vi "DataSelect.vi"(8 "error in (no error)":errorcluster, 10 "Table":string, 11 "Machine":string) -> (0 "error out":errorcluster)   [LabVIEW 2012]
uses:
  <vilib>/addons/database/Connection.llb/DB Tools Open Connec (Path).vi
  <vilib>/addons/database/_DB Variant To Data/Database Variant To Data.xnode
  <vilib>/addons/database/NI_Database_API.lvlib
panel:
  out "data 2":string
  out "element":i32
  out "x = y? 2":bool
  out "sum":i32
  out "concatenated string 2":string
  out "output cluster 2":T1
  in  "input cluster 2":T1
  out "sum 2":i32
  out "x = y?":bool
  out "output cluster":T1
  in  "input cluster":T1
  out "data":variant[][](array[variant])
  out "concatenated string":string
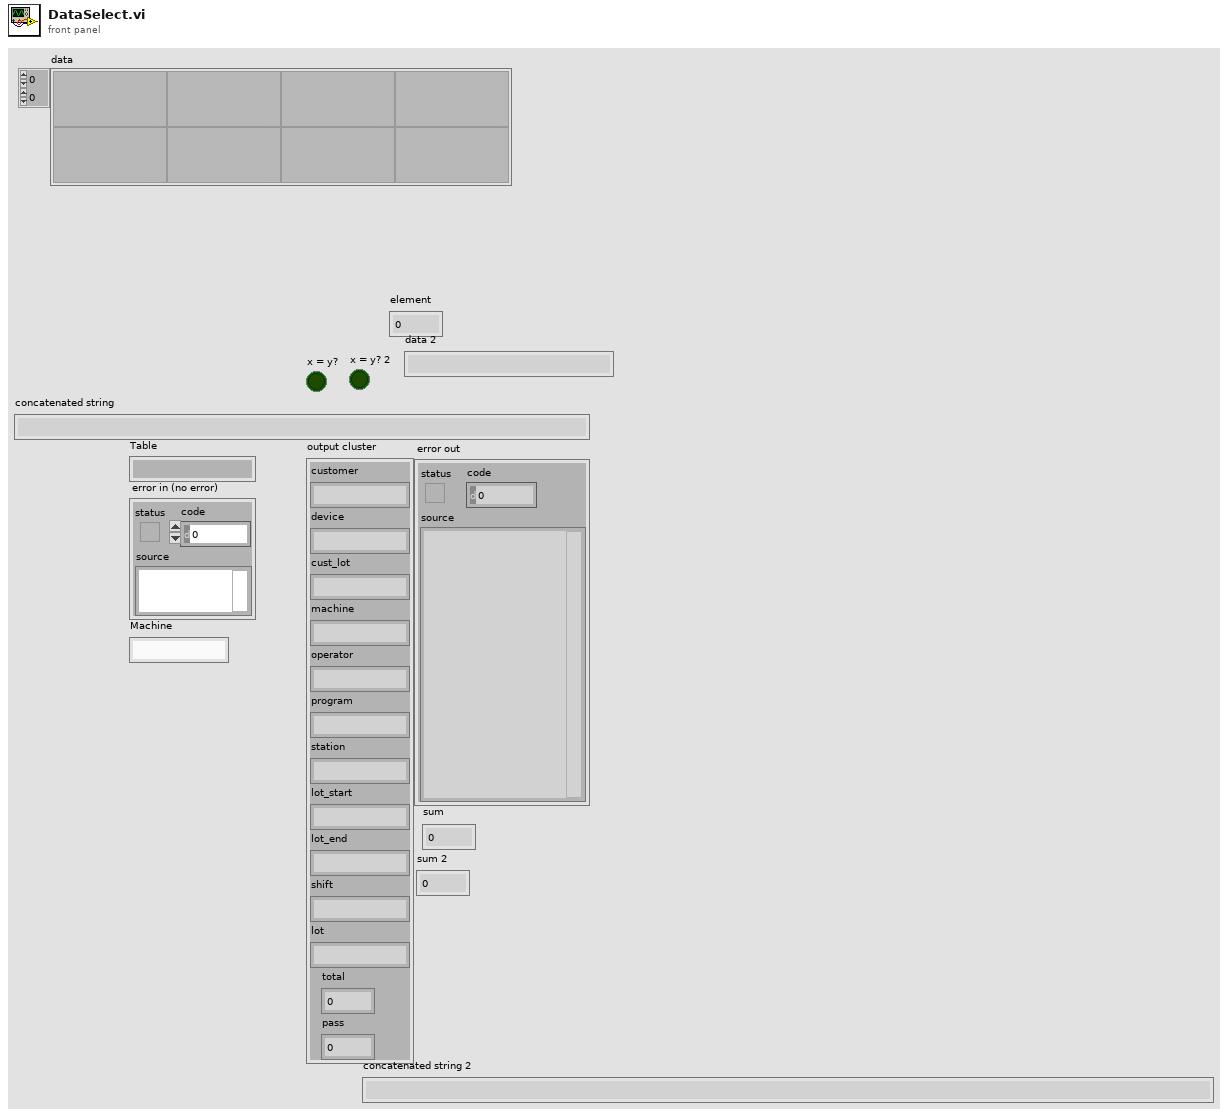
[diagram p1: front panel]
types:
  T1 = cluster{"customer":string, "device":string, "cust_lot":string, "machine":string, "operator":string, "program":string, "station":string, "lot_start":string, "lot_end":string, "shift":string, "lot":string, "total":dbl, "pass":dbl}
  T2 = typedef "NI_Database_API.lvlib/Conn ObjectReference.ctl" = refnum<k1>
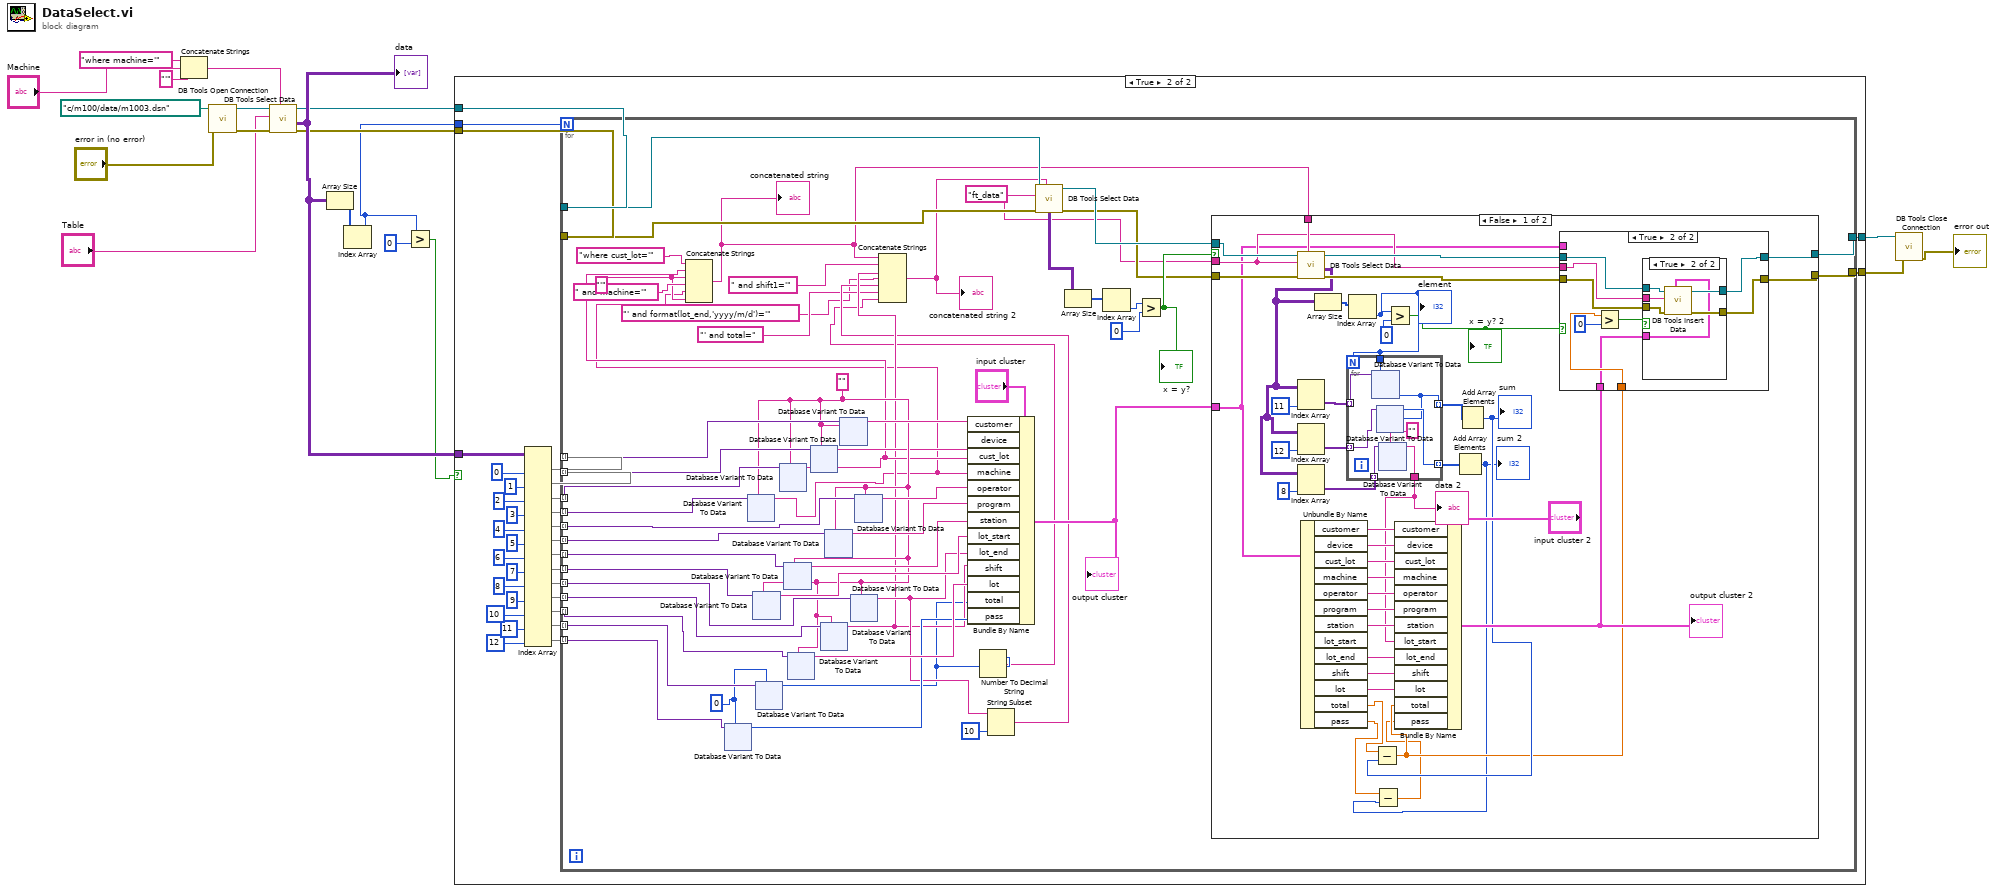
[diagram p0: block diagram]
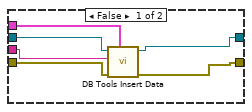
[diagram p3: hidden frame]
diagram:
  n1 = Concatenate Strings("where machine='" ("string"), "Machine", "'" ("string")) -> (w6:string)
  n2 = call-poly <vilib>:"DB Tools Open Connection.vi"("error in (no error)"="error in (no error)", "connection information"=path "c:/m100/data/m1003.dsn") -> ("error out"=w17:errorcluster, "connection reference"=w18:T2)  [unwired: 6 in]
  n3 = call <vilib>:"DB Tools Select Data.vi"("condition"=w6, "error in (no error)"=w17, "table"="Table", "connection reference"=w18) -> ("error out"=w3:errorcluster, "data"=w15:variant[][], "connection reference out"=w4:T2)  [unwired: 2 in]
  "data" <- w15
  n4 = Array Size(array=w15) -> (size(s)=w16:i32[])
  n5 = Index Array(array=w16) -> (element=w2:i32)  [unwired: 1 in]
  n6 = Greater?(x=w2, y=0) -> (0:w1:bool)
  n7 = case shown="True" w1 {
    tunnel: w15 -> [_ w52]
    tunnel: [w21 w26] -> w14
    tunnel: [w20 w25] -> w13
    tunnel: w4 -> [w21 w24]
    tunnel: w3 -> [w20 w23]
    tunnel: w2 -> [_ w22]
    frame False {
    }
    frame True {
      n8 = Index Array(array=w52, index (col) #1=0 ("disabled index (col)"), index (col) #2=1 ("index (col)"), index (col) #3=2 ("index (col)"), index (col) #4=3 ("index (col)"), index (col) #5=4 ("index (col)"), index (col) #6=5 ("index (col)"), index (col) #7=6 ("index (col)"), index (col) #8=7 ("index (col)"), index (col) #9=8 ("index (col)"), index (col) #10=9 ("index (col)"), index (col) #11=10 ("index (col)"), index (col) #12=11 ("index (col)"), index (col) #13=12 ("index (col)")) -> (element #1=w39:variant[], element #2=w38:variant[], element #3=w37:variant[], element #4=w36:variant[], element #5=w35:variant[], element #6=w34:variant[], element #7=w33:variant[], element #8=w32:variant[], element #9=w31:variant[], element #10=w30:variant[], element #11=w29:variant[], element #12=w28:variant[], element #13=w27:variant[])  [unwired: 13 in]
      n9 = for {
        N: w22 -> [_]
        tunnel: w24 -> [w83]
        tunnel: w23 -> [w82]
        tunnel: w39 -> [w105] mode=indexing
        tunnel: w38 -> [w104] mode=indexing
        tunnel: w37 -> [w103] mode=indexing
        tunnel: w36 -> [w102] mode=indexing
        tunnel: w35 -> [w92] mode=indexing
        tunnel: w34 -> [w101] mode=indexing
        tunnel: w33 -> [w100] mode=indexing
        tunnel: w32 -> [w99] mode=indexing
        tunnel: w31 -> [w98] mode=indexing
        tunnel: w30 -> [w97] mode=indexing
        tunnel: w29 -> [w96] mode=indexing
        tunnel: w28 -> [w95] mode=indexing
        tunnel: w27 -> [w94] mode=indexing
        tunnel: [w71] -> w26
        tunnel: [w70] -> w25
        w56 = "'" ("string")
        w73 = "ft_data" ("table")
        w93 = 0
        w79 = ""
        n10 = xnode "Database Variant To Data"("database variant"=w94, "type"=w93) -> ("data"=w85:i32)  [unwired: 1 in, 1 out]
        n11 = xnode "Database Variant To Data"("database variant"=w102, "type"=w79) -> ("data"=w55:string)  [unwired: 1 in, 1 out]
        n12 = xnode "Database Variant To Data"("database variant"=w99, "type"=w79) -> ("data"=w87:string)  [unwired: 1 in, 1 out]
        n13 = xnode "Database Variant To Data"("database variant"=w95, "type"=w93) -> ("data"=w61:i32)  [unwired: 1 in, 1 out]
        n14 = xnode "Database Variant To Data"("database variant"=w103, "type"=w79) -> ("data"=w67:string)  [unwired: 1 in, 1 out]
        n15 = Concatenate Strings("where cust_lot='" ("string"), w67, w56, " and machine='" ("string"), w55, w56) -> (w54:string)
        "concatenated string" <- w54
        n16 = xnode "Database Variant To Data"("database variant"=w100, "type"=w79) -> ("data"=w88:string)  [unwired: 1 in, 1 out]
        n17 = xnode "Database Variant To Data"("database variant"=w96, "type"=w79) -> ("data"=w86:string)  [unwired: 1 in, 1 out]
        n18 = xnode "Database Variant To Data"("database variant"=w104, "type"=w79) -> ("data"=w68:string)  [unwired: 1 in, 1 out]
        n19 = xnode "Database Variant To Data"("database variant"=w97, "type"=w79) -> ("data"=w64:string)  [unwired: 1 in, 1 out]
        n20 = xnode "Database Variant To Data"("database variant"=w101, "type"=w79) -> ("data"=w89:string)  [unwired: 1 in, 1 out]
        n21 = xnode "Database Variant To Data"("database variant"=w105, "type"=w79) -> ("data"=w91:string)  [unwired: 1 in, 1 out]
        n22 = xnode "Database Variant To Data"("database variant"=w98, "type"=w79) -> ("data"=w77:string)  [unwired: 1 in, 1 out]
        n23 = xnode "Database Variant To Data"("database variant"=w92, "type"=w79) -> ("data"=w90:string)  [unwired: 1 in, 1 out]
        n24 = Bundle By Name(cluster="input cluster", "customer"=w91, "device"=w68, "cust_lot"=w67, "machine"=w55, "operator"=w90, "program"=w89, "station"=w88, "lot_start"=w87, "lot_end"=w77, "shift"=w64, "lot"=w86, "total"=w61, "pass"=w85) -> (w72:T1)
        "output cluster" <- w72
        n25 = Number To Decimal String(number=w61) -> (decimal integer string=w59:string)  [unwired: 1 in]
        n26 = String Subset(string=w77, length (rest)=10 ("length (rest)")) -> (substring=w63:string)  [unwired: 1 in]
        n27 = Concatenate Strings(w54, " and shift1='" ("string"), w64, "' and format(lot_end,'yyyy/m/d')='" ("string"), w63, "' and total=" ("string"), w59) -> (w58:string)
        "concatenated string 2" <- w58
        n28 = call <vilib>:"DB Tools Select Data.vi"("condition"=w58, "error in (no error)"=w82, "table"=w73, "connection reference"=w83) -> ("error out"=w74:errorcluster, "data"=w81:variant[][], "connection reference out"=w75:T2)  [unwired: 2 in]
        n29 = Array Size(array=w81) -> (size(s)=w80:i32[])
        n30 = Index Array(array=w80) -> (element=w69:i32)  [unwired: 1 in]
        n31 = Greater?(x=w69, y=0) -> (0:w76:bool)
        "x = y?" <- w76
        n32 = case shown="False" w76 {
          tunnel: w75 -> [w147 w276]
          tunnel: w74 -> [w146 w275]
          tunnel: w73 -> [w119 _]
          tunnel: w72 -> [w118 _]
          tunnel: [w137 w276] -> w71
          tunnel: [w136 w275] -> w70
          tunnel: w54 -> [w121 _]
          frame False {
            n33 = call <vilib>:"DB Tools Select Data.vi"("condition"=w121, "error in (no error)"=w146, "table"=w119, "connection reference"=w147) -> ("error out"=w142:errorcluster, "data"=w111:variant[][], "connection reference out"=w143:T2)  [unwired: 2 in]
            n34 = Index Array(array=w111, index (col)=11) -> (element=w139:variant[])  [unwired: 1 in]
            n35 = Index Array(array=w111, index (col)=12) -> (element=w133:variant[])  [unwired: 1 in]
            n36 = Index Array(array=w111, index (col)=8 ("disabled index (col)")) -> (element=w108:variant[])  [unwired: 1 in]
            n37 = Unbundle By Name(w118) -> ("customer"=w109:string, "device"=w131:string, "cust_lot"=w130:string, "machine"=w129:string, "operator"=w128:string, "program"=w127:string, "station"=w126:string, "lot_end"=w125:string, "shift"=w124:string, "lot"=w123:string, "total"=w117:dbl, "pass"=w114:dbl)  [unwired: 1 out]
            n38 = Array Size(array=w111) -> (size(s)=w145:i32[])
            n39 = Index Array(array=w145) -> (element=w138:i32)  [unwired: 1 in]
            "element" <- w138
            n40 = for {
              N: w138 -> [_]
              tunnel: w139 -> [w155] mode=indexing
              tunnel: w138 -> [w154]
              tunnel: [w151] -> w135 mode=indexing
              tunnel: w133 -> [w153] mode=indexing
              tunnel: [w152] -> w132 mode=indexing
              tunnel: w108 -> [w150] mode=indexing
              tunnel: [w148] -> w107
              n41 = xnode "Database Variant To Data"("database variant"=w155, "type"=w154) -> ("data"=w151:i32)  [unwired: 1 in, 1 out]
              n42 = xnode "Database Variant To Data"("database variant"=w153, "type"=w151) -> ("data"=w152:i32)  [unwired: 1 in, 1 out]
              n43 = xnode "Database Variant To Data"("database variant"=w150, "type"="") -> ("data"=w148:string)  [unwired: 1 in, 1 out]
            }
            "data 2" <- w107
            n44 = Greater?(x=w138, y=0) -> (0:w144:bool)
            "x = y? 2" <- w144
            n45 = Add Array Elements(numeric array=w132) -> (sum=w113:i32)
            "sum 2" <- w113
            n46 = Subtract(x=w114, y=w113) -> (x-y=w112:dbl)
            n47 = Add Array Elements(numeric array=w135) -> (sum=w116:i32)
            "sum" <- w116
            n48 = Subtract(x=w117, y=w116) -> (x-y=w115:dbl)
            n49 = Bundle By Name(cluster="input cluster 2", "customer"=w109, "device"=w131, "cust_lot"=w130, "machine"=w129, "operator"=w128, "program"=w127, "station"=w126, "lot_start"=w107, "lot_end"=w125, "shift"=w124, "lot"=w123, "total"=w115, "pass"=w112) -> (w120:T1)
            "output cluster 2" <- w120
            n50 = case shown="True" w144 {
              tunnel: w143 -> [w257 w263]
              tunnel: w142 -> [w256 w262]
              tunnel: [w255 w260] -> w137
              tunnel: [w254 w259] -> w136
              tunnel: w120 -> [_ w258]
              tunnel: w119 -> [w253 w261]
              tunnel: w118 -> [w252 _]
              tunnel: w115 -> [_ w265]
              frame False {
                n51 = call <vilib>:"DB Tools Insert Data.vi"("data"=w252, "error in (no error)"=w256, "table"=w253, "connection reference"=w257) -> ("error out"=w254:errorcluster, "connection reference out"=w255:T2)  [unwired: 6 in]
              }
              frame True {
                n52 = Greater?(x=w265, y=0) -> (0:w264:bool)
                n53 = case shown="True" w264 {
                  tunnel: w263 -> [w268 w274]
                  tunnel: w262 -> [w267 w273]
                  tunnel: w261 -> [_ w272]
                  tunnel: [w268 w271] -> w260
                  tunnel: [w267 w270] -> w259
                  tunnel: w258 -> [_ w269]
                  frame False {
                  }
                  frame True {
                    n54 = call <vilib>:"DB Tools Insert Data.vi"("data"=w269, "error in (no error)"=w273, "table"=w272, "connection reference"=w274) -> ("error out"=w270:errorcluster, "connection reference out"=w271:T2)  [unwired: 6 in]
                  }
                }
              }
            }
          }
          frame True {
          }
        }
      }
    }
  }
  n55 = call <vilib>:"DB Tools Close Connection.vi"("error in (no error)"=w13, "connection reference"=w14) -> ("error out"=→"error out":errorcluster)  [unwired: 5 in]
